vi "ASIA Release Pump.vi"(8 "error in (no error)":errorcluster, 11 "pumpNum":u32) -> (0 "error out":errorcluster, 3 "ASIA Pump # Out":i32)   [LabVIEW 2018, in "ASIA Pump.lvlib"]
uses:
  ASIA Pump.lvlib
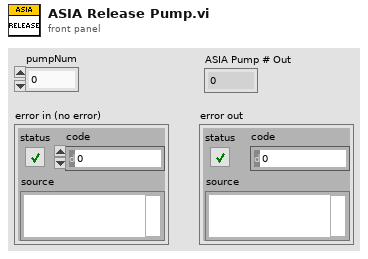
[diagram p1: front panel]
types:
  T1 = cluster{"Busy":bool, "PumpCnt":dbl, "RemoteEntered":bool, "OverpressureSet":bool}[]
  T2 = cluster{"Busy":bool, "PumpCnt":dbl, "RemoteEntered":bool, "OverpressureSet":bool}
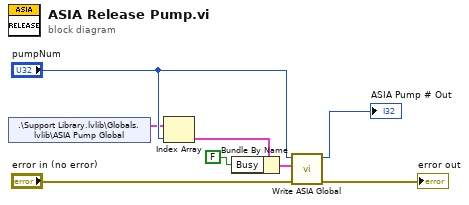
[diagram p0: block diagram]
diagram:
  n1 = shared-variable ".\\Support Library.lvlib\\Globals.lvlib\\ASIA Pump Global"() -> (w2:T1)  [unwired: 1 in, 1 out]
  n2 = Index Array(array=w2, index="pumpNum") -> (element=w3:T2)
  n3 = Bundle By Name(cluster=w3, "Busy"=FALSE) -> (w6:T2)
  n4 = call "Write ASIA Global.vi"("error in (no error)"="error in (no error)", "ASIA Global"=w6, "Pump Number In"="pumpNum") -> ("error out"=→"error out":errorcluster, "Pump Number Out"=→"ASIA Pump # Out":i32)  [unwired: 7 in]
